vi "Read Report Details.vi"(8 "error in (no error)":errorcluster, 11 "Report in":refnum<class "Report.lvclass">) -> (0 "error out":errorcluster, 2 "Report Details":T1, 3 "Report out":refnum<class "Report.lvclass">)   [LabVIEW 2019, in "Report.lvlib" / "Report.lvclass"]
uses:
  Report.lvclass
  Report.lvclass/Report.ctl
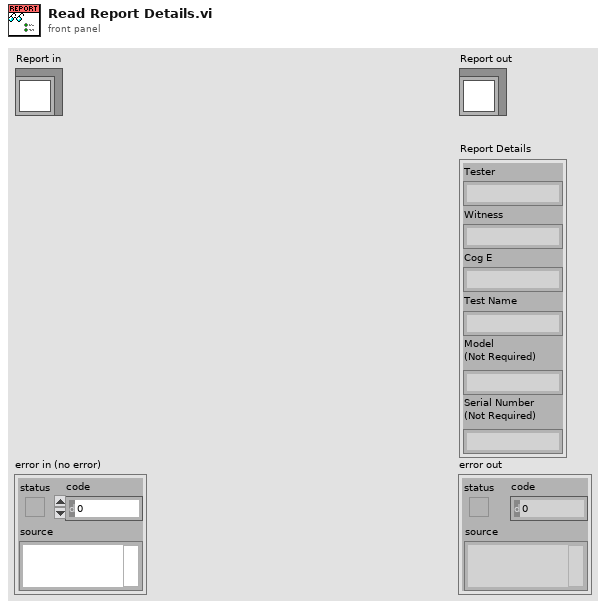
[diagram p1: front panel]
types:
  T1 = cluster{"Tester":string, "Witness":string, "Cog E":string, "Test Name":string, "Model\n(Not Required)":string, "Serial Number\n(Not Required)":string}
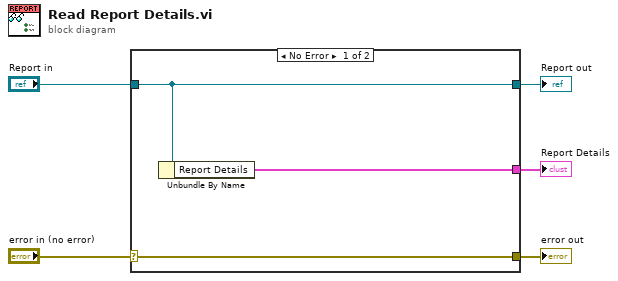
[diagram p0: block diagram]
diagram:
  n1 = case shown="No Error" "error in (no error)" {
    selector: "error in (no error)" -> [w8 w9]
    tunnel: [w8 w9] -> w4
    tunnel: [w7 w10] -> w2
    tunnel: "Report in" -> [w7 w10]
    tunnel: [w6 _] -> w1
    frame No Error {
      n2 = Unbundle By Name(w7) -> ("Report Details"=w6:T1)
    }
    frame Error {
    }
  }
  "error out" <- w4
  "Report out" <- w2
  "Report Details" <- w1
